vi "VMI_set_file_date.vi"(0 "Saved date":string="110416", 1 "Ending":string="aa") -> (2 "New Date Name":string, 3 "New Date":string, 4 "New letters":string)   [LabVIEW 2018]
panel:
  out "unsigned byte array":u8[](array[numeric])
  out "x = y?":bool
  out "Stripped String":string
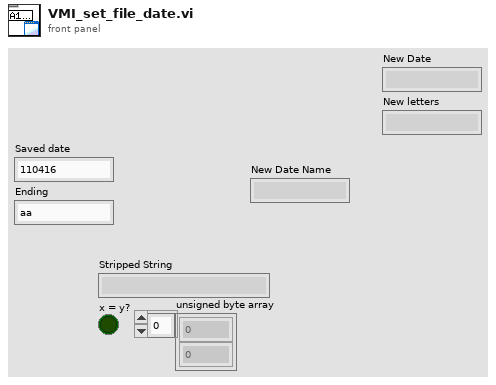
[diagram p1: front panel]
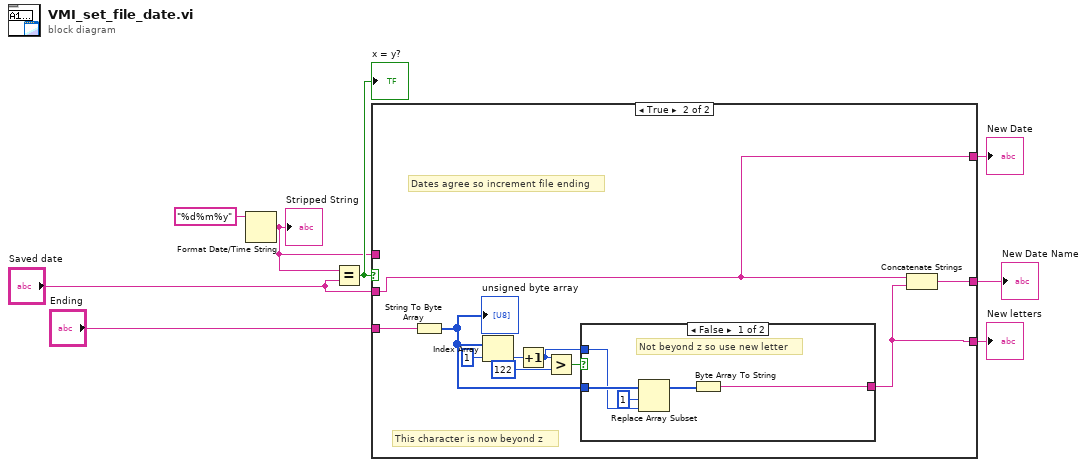
[diagram p0: block diagram]
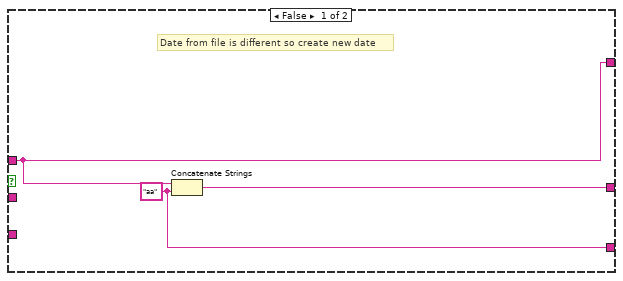
[diagram p2: hidden frame]
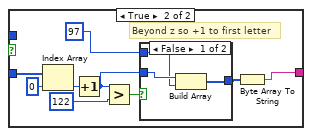
[diagram p3: hidden frame]
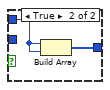
[diagram p4: hidden frame]
diagram:
  n1 = Format Date/Time String(time format string (%c)="%d%m%y") -> (date/time string=w6:string)  [unwired: 2 in]
  "Stripped String" <- w6
  n2 = Equal?(x=w6, y="Saved date") -> (x = y?=w7:bool)
  "x = y?" <- w7
  n3 = case shown="True" w7 {
    tunnel: w6 -> [w10 _]
    tunnel: [w11 w14] -> w3
    tunnel: "Saved date" -> [_ w13]
    tunnel: "Ending" -> [_ w21]
    tunnel: [w10 w13] -> w2
    tunnel: [w9 w12] -> w1
    frame False {
      w9 = "aa" ("string")
      # "Date from file is different so create new date"
      n4 = Concatenate Strings(w10, w9) -> (w11:string)
    }
    frame True {
      # "This character is now beyond z"
      # "Dates agree so increment file ending"
      n5 = String To Byte Array(string=w21) -> (unsigned byte array=w16:u8[])
      "unsigned byte array" <- w16
      n6 = Index Array(array=w16, index=1) -> (element=w19:u8)
      n7 = Increment(x=w19) -> (x+1=w15:u8)
      n8 = Greater?(x=w15, y=u8 122) -> (0:w17:bool)
      n9 = case shown="False" w17 {
        tunnel: w16 -> [w26 w29]
        tunnel: w15 -> [w24 _]
        tunnel: [w22 w28] -> w12
        frame False {
          # "Not beyond z so use new letter"
          n10 = Replace Array Subset(array=w26, new element=w24, index=1) -> (w23:u8[])
          n11 = Byte Array To String(unsigned byte array=w23) -> (string=w22:string)
        }
        frame True {
          # "Beyond z so +1 to first letter"
          n12 = Index Array(array=w29, index=0) -> (element=w34:u8)
          n13 = Increment(x=w34) -> (x+1=w31:u8)
          n14 = Greater?(x=w31, y=u8 122) -> (0:w32:bool)
          n15 = case shown="False" w32 {
            tunnel: w31 -> [w38 _]
            tunnel: 97 -> [w37 w40]
            tunnel: [w36 w39] -> w27
            frame False {
              n16 = Build Array(w38, w37) -> (w36:i32[])
            }
            frame True {
              n17 = Build Array(w40, w40) -> (w39:i32[])
            }
          }
          n18 = Byte Array To String(unsigned byte array=w27) -> (string=w28:string)
        }
      }
      n19 = Concatenate Strings(w13, w12) -> (w14:string)
    }
  }
  "New Date Name" <- w3
  "New Date" <- w2
  "New letters" <- w1
